vi "Kernel - Data Acquisition.vi"(7 "Cluster":T1={"Count (uSec)"=0, "Timed Out?"=FALSE, "Samples per Channel"=2000}, 8 "error in":errorcluster, 10 "State":string, 11 "message queue":refnum<queue>) -> (0 "error out":errorcluster, 3 "message queue (out)":refnum<queue>, 4 "Stop?":bool, 5 "Cluster 2":T1={"Count (uSec)"=0, "Timed Out?"=FALSE, "Samples per Channel"=2000})   [LabVIEW 2021]
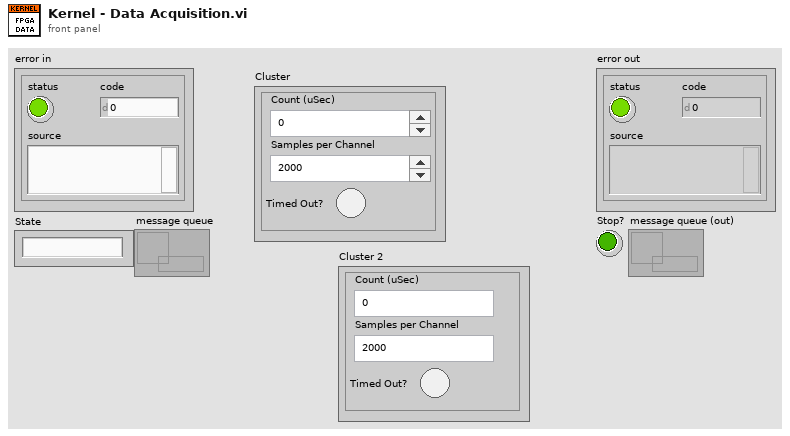
[diagram p1: front panel]
types:
  T1 = cluster{"Count (uSec)":i32, "Timed Out?":bool, "Samples per Channel":i32}
  T2 = typedef "Data - Error Handler.ctl" = cluster{"message queues":refnum<queue>[], "queue reference - error handler":refnum<queue>, "error":errorcluster}
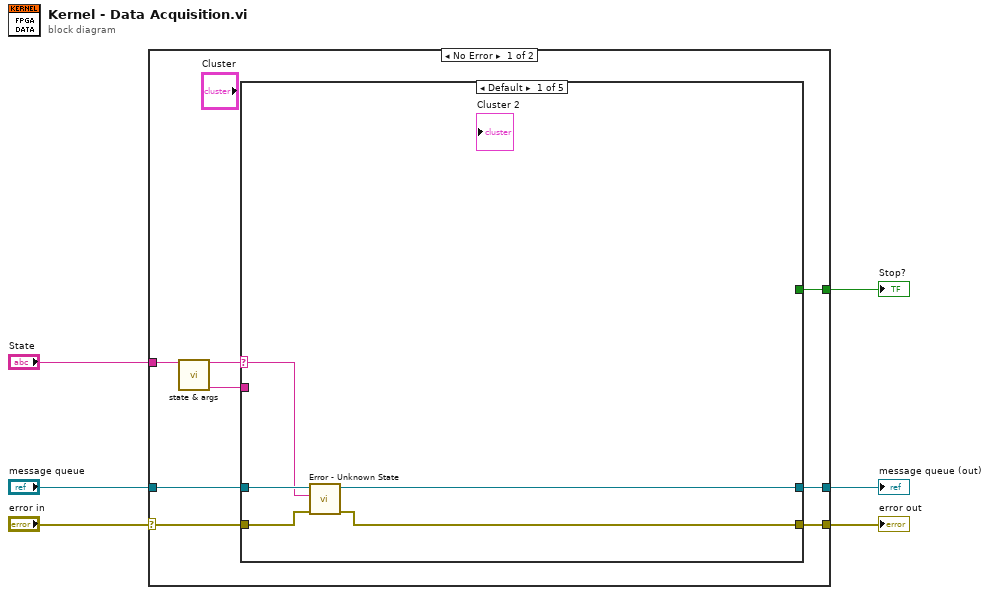
[diagram p0: block diagram]
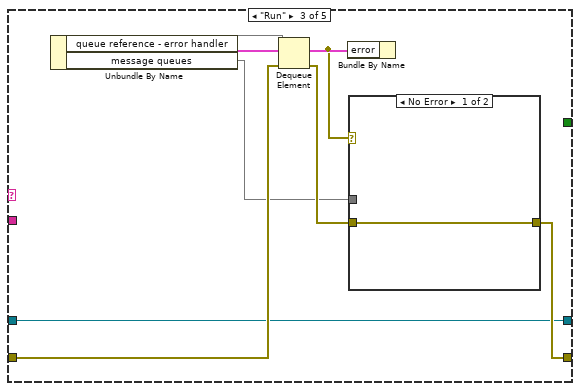
[diagram p3: hidden frame]
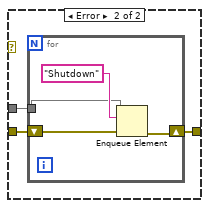
[diagram p4: hidden frame]
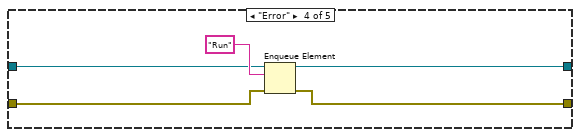
[diagram p5: hidden frame]
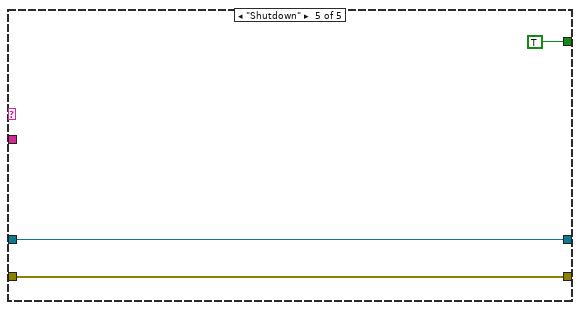
[diagram p6: hidden frame]
diagram:
  n1 = case shown="No Error" "error in" {
    selector: "error in" -> [w10 w47]
    tunnel: "State" -> [w14 _]
    tunnel: "message queue" -> [w11 w48]
    tunnel: [w9 w48] -> w3
    tunnel: [w8 w47] -> w2
    tunnel: [w7 _] -> w1
    frame No Error {
      n2 = call "state & args.vi"("state:args"=w14) -> ("args"=w12:string, "state"=w13:string)  [unwired: 9 in]
      n3 = case shown="Default" w13 {
        selector: w13 -> [w17 _ _ _ _]
        tunnel: w12 -> [_ _ _ _ _]
        tunnel: w11 -> [w19 w21 w22 w41 w45]
        tunnel: w10 -> [w18 w20 w29 w40 w44]
        tunnel: [w16 w21 w22 w42 w45] -> w9
        tunnel: [w15 w20 w23 w39 w44] -> w8
        tunnel: [_ _ _ _ TRUE] -> w7
        frame Default {
          n4 = call "Error - Unknown State.vi"("error in"=w18, "state"=w17, "queue"=w19) -> ("error out"=w15:errorcluster, "queue out"=w16:refnum<queue>)  [unwired: 7 in]
        }
        frame "Initialize" {
        }
        frame "Run" {
          n5 = Unbundle By Name() -> (w28:T2, "queue reference - error handler"=w30, "message queues"=w24)
          n6 = Dequeue Element(queue=w30, error in (no error)=w29) -> (element=w26:errorcluster, error out=w25:errorcluster)  [unwired: 1 in, 2 out]
          n7 = Bundle By Name(cluster=w28, "error"=w26) -> (w27:cluster{})
          n8 = case shown="No Error" w26 {
            tunnel: w25 -> [w31 w34]
            tunnel: w24 -> [_ w32]
            tunnel: [w31 w33] -> w23
            frame No Error {
            }
            frame Error {
              n9 = for {
                shift-right: [w37] -> w33
                shift-left: w34 -> [w38]
                tunnel: w32 -> [w35]
                n10 = Enqueue Element(queue=w35, element="Shutdown", error in (no error)=w38) -> (error out=w37:errorcluster)  [unwired: 1 in, 2 out]
              }
            }
          }
        }
        frame "Error" {
          n11 = Enqueue Element(queue=w41, element="Run", error in (no error)=w40) -> (queue out=w42:refnum<queue>, error out=w39:errorcluster)  [unwired: 1 in, 1 out]
        }
        frame "Shutdown" {
        }
      }
    }
    frame Error {
    }
  }
  "error out" <- w2
  "Stop?" <- w1
  "message queue (out)" <- w3
